vi "Application_GetTimeInError.vi"(10 "Errorin":errorcluster) -> (2 "Errorout":errorcluster, 3 "relative seconds":dbl)   [LabVIEW 2016]
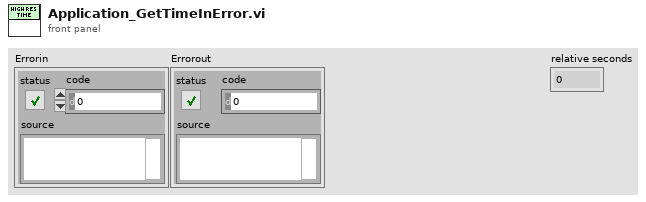
[diagram p1: front panel]
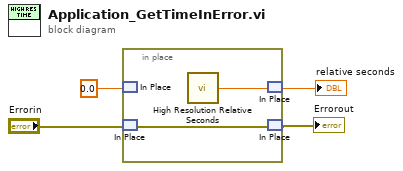
[diagram p0: block diagram]
diagram:
  n1 = in-place {
    n2 = in-place-match #1(0.0 ("relative seconds")) -> ()  [unwired: 1 out]
    n3 = in-place-match #2("Errorin") -> (w6:errorcluster)
    n4 = call <vilib>:"High Resolution Relative Seconds.vi"() -> ("relative seconds"=w5:dbl)
    n5 = in-place-match #1(w5) -> (→"relative seconds":dbl)
    n6 = in-place-match #2(w6) -> (→"Errorout":errorcluster)
  }
